vi "ZK HAL.vi"(11 "Interface":T1={"SYSTEM Interface"={"运行模式"=enum."维护模式", "站点类型"=enum."一体站", "CODMn类型"=enum."PLC版", "总磷总氮类型"=enum."单模块"}, "Pump Interface"={"Pump MB session in"=refnum}, "NH3N Interface"={"NH3N session in"=refnum, "氨氮自动测试量程配置"={"水样测试量程模式"=enum."AUTO", "空白核查量程模式"=enum."AUTO", "跨度核查量程模式"=enum."AUTO", "加标回收量程模式"=enum."AUTO"}}, "TP Interface"={"TP MB session in"=refnum, "总磷自动测试量程配置"={"水样测试量程模式"=enum."AUTO", "空白核查量程模式"=enum."AUTO", "跨度核查量程模式"=enum."AUTO", "加标回收量程模式"=enum."AUTO"}}, "TN Interface"={"TN MB session in"=refnum, "总氮自动测试量程配置"={"水样测试量程模式"=enum."AUTO", "空白核查量程模式"=enum."AUTO", "跨度核查量程模式"=enum."AUTO", "加标回收量程模式"=enum."AUTO"}}, "CODMn Interface"={"CODMn MB session in"=refnum, "CODMn自动测试量程配置"={"水样测试量程模式"=enum."AUTO", "空白核查量程模式"=enum."AUTO", "跨度核查量程模式"=enum."AUTO", "加标回收量程模式"=enum."AUTO"}}, "CODCr Interface"={"CODCr MB session in"=refnum, "CODCr自动测试量程配置"={"水样测试量程模式"=enum."AUTO", "空白核查量程模式"=enum."AUTO", "跨度核查量程模式"=enum."AUTO", "加标回收量程模式"=enum."AUTO"}}, "PLC_CODMn Interface"={"PLC版_CODMn状态"=0, "PLC版_CODMn测量数据区"={"因子编码"=0, "单位"=0, "标样参考值"=0.0, "水样数据时间"=timestamp(0 s since 1904-01-01), "水样实测值"=0.0, "水样数据标识"="", "标样数据时间"=timestamp(0 s since 1904-01-01), "标样实测值"=0.0, "标样数据标识"="", "空白数据时间"=timestamp(0 s since 1904-01-01), "空白实测值"=0.0, "空白数据标识"="", "零点核查数据时间"=timestamp(0 s since 1904-01-01), "零点核查实测值"=0.0, "零点核查数据标识"="", "跨度核查数据时间"=timestamp(0 s since 1904-01-01), "跨度核查实测值"=0.0, "跨度核查数据标识"="", "加标回收数据时间"=timestamp(0 s since 1904-01-01), "加标回收实测值"=0.0, "加标回收数据标识"="", "平行样数据时间"=timestamp(0 s since 1904-01-01), "平行样实测值"=0.0, "平行样数据标识"=""}}} {"PLC_CODMn Interface"."PLC版_CODMn状态" items=["待机", "润洗", "进样", "加草酸钠", "反滴定", "排液"]; "PLC_CODMn Interface"."PLC版_CODMn测量数据区"."单位" items=["ug/L", "mg/L", "ppm", "mg/m3", "cm", "ppb", "ug/m3", "%", "nmol/mol", "umol/mol", "MPN/L", "MPN/100ml", "ng/m3", "NTU", "无量纲", "ms/cm", "us/cm", "℃", "mV", "万个/L"]}) -> ()   [LabVIEW 2016]
uses:
  <vilib>/Plasmionique/MB Master/MB_Master/MB_Master.lvclass
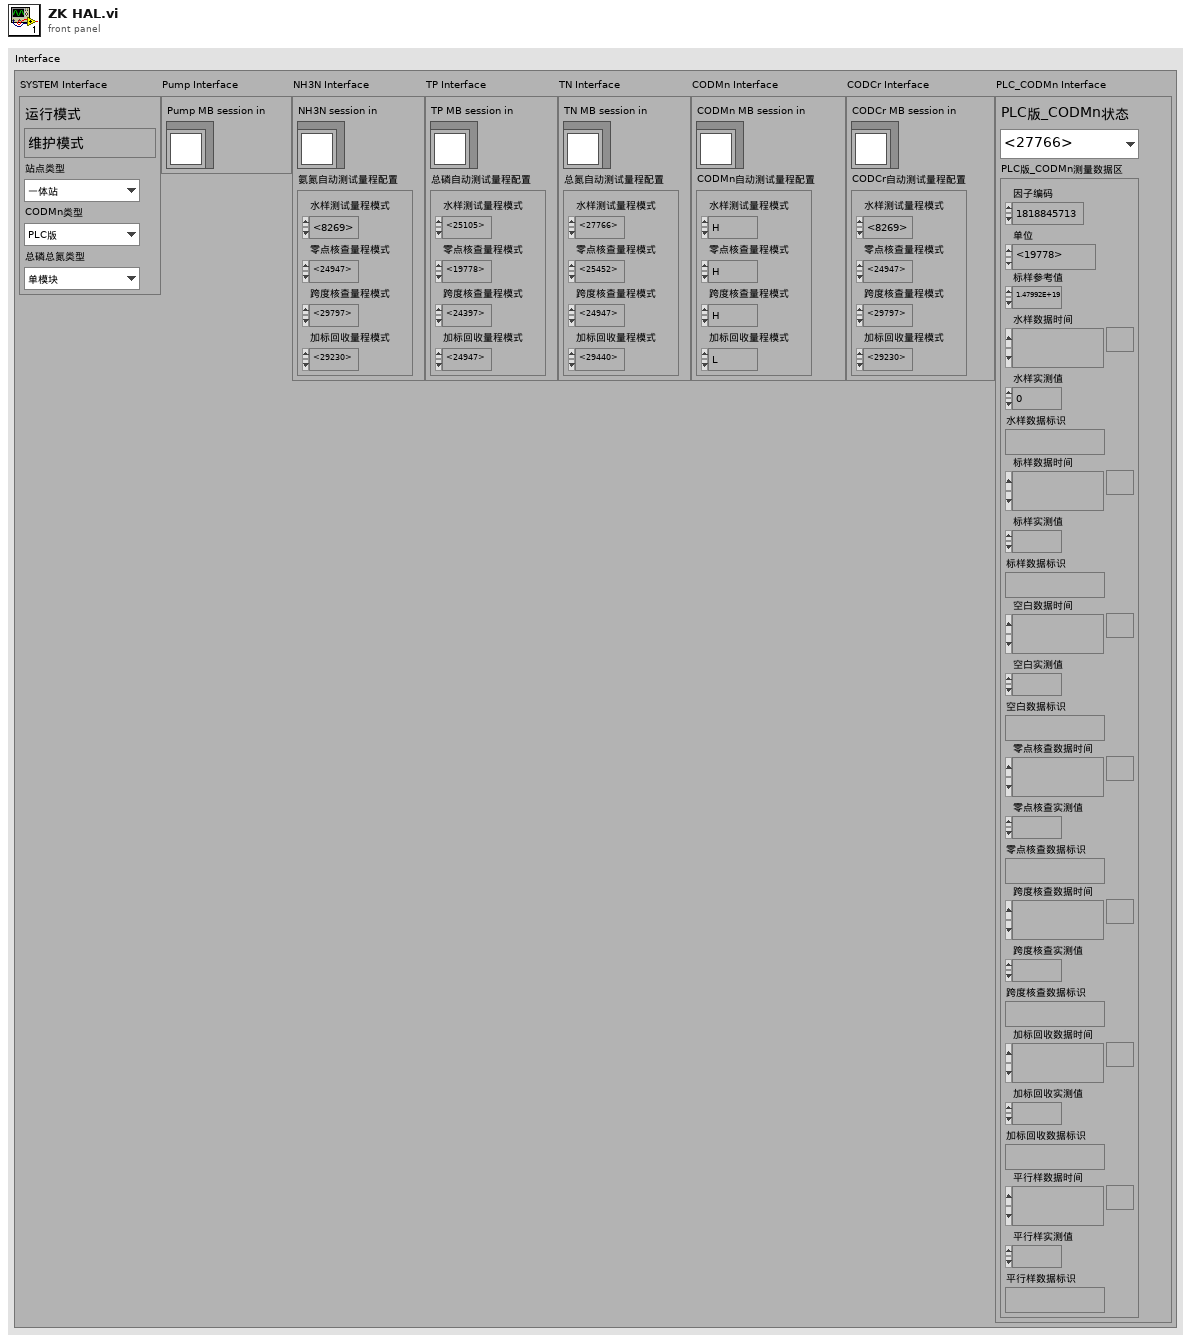
[diagram p1: front panel]
types:
  T1 = cluster{"SYSTEM Interface":cluster{"运行模式":enum16{"维护模式", "常规模式", "应急模式", "质控模式"}, "站点类型":enum16{"一体站", "固定站", "浮船"}, "CODMn类型":enum16{"PLC版", "单片机版"}, "总磷总氮类型":enum16{"单模块", "二合一模块"}}, "Pump Interface":cluster{"Pump MB session in":refnum<class "MB_Master.lvclass">}, "NH3N Interface":cluster{"NH3N session in":refnum<class "MB_Master.lvclass">, "氨氮自动测试量程配置":cluster{"水样测试量程模式":enum16{"H", "L", "AUTO"}, "空白核查量程模式":enum16{"H", "L", "AUTO"}, "跨度核查量程模式":enum16{"H", "L", "AUTO"}, "加标回收量程模式":enum16{"H", "L", "AUTO"}}}, "TP Interface":cluster{"TP MB session in":refnum<class "MB_Master.lvclass">, "总磷自动测试量程配置":cluster{"水样测试量程模式":enum16{"H", "L", "AUTO"}, "空白核查量程模式":enum16{"H", "L", "AUTO"}, "跨度核查量程模式":enum16{"H", "L", "AUTO"}, "加标回收量程模式":enum16{"H", "L", "AUTO"}}}, "TN Interface":cluster{"TN MB session in":refnum<class "MB_Master.lvclass">, "总氮自动测试量程配置":cluster{"水样测试量程模式":enum16{"H", "L", "AUTO"}, "空白核查量程模式":enum16{"H", "L", "AUTO"}, "跨度核查量程模式":enum16{"H", "L", "AUTO"}, "加标回收量程模式":enum16{"H", "L", "AUTO"}}}, "CODMn Interface":cluster{"CODMn MB session in":refnum<class "MB_Master.lvclass">, "CODMn自动测试量程配置":cluster{"水样测试量程模式":enum16{"H", "L", "AUTO"}, "空白核查量程模式":enum16{"H", "L", "AUTO"}, "跨度核查量程模式":enum16{"H", "L", "AUTO"}, "加标回收量程模式":enum16{"H", "L", "AUTO"}}}, "CODCr Interface":cluster{"CODCr MB session in":refnum<class "MB_Master.lvclass">, "CODCr自动测试量程配置":cluster{"水样测试量程模式":enum16{"H", "L", "AUTO"}, "空白核查量程模式":enum16{"H", "L", "AUTO"}, "跨度核查量程模式":enum16{"H", "L", "AUTO"}, "加标回收量程模式":enum16{"H", "L", "AUTO"}}}, "PLC_CODMn Interface":cluster{"PLC版_CODMn状态":u16, "PLC版_CODMn测量数据区":cluster{"因子编码":u32, "单位":u16, "标样参考值":sgl, "水样数据时间":timestamp, "水样实测值":sgl, "水样数据标识":string, "标样数据时间":timestamp, "标样实测值":sgl, "标样数据标识":string, "空白数据时间":timestamp, "空白实测值":sgl, "空白数据标识":string, "零点核查数据时间":timestamp, "零点核查实测值":sgl, "零点核查数据标识":string, "跨度核查数据时间":timestamp, "跨度核查实测值":sgl, "跨度核查数据标识":string, "加标回收数据时间":timestamp, "加标回收实测值":sgl, "加标回收数据标识":string, "平行样数据时间":timestamp, "平行样实测值":sgl, "平行样数据标识":string}}}
  T2 = cluster{"运行模式":enum16{"维护模式", "常规模式", "应急模式", "质控模式"}, "站点类型":enum16{"一体站", "固定站", "浮船"}, "CODMn类型":enum16{"PLC版", "单片机版"}, "总磷总氮类型":enum16{"单模块", "二合一模块"}}
  T3 = cluster{"Pump MB session in":refnum<class "MB_Master.lvclass">}
  T4 = cluster{"NH3N session in":refnum<class "MB_Master.lvclass">, "氨氮自动测试量程配置":cluster{"水样测试量程模式":enum16{"H", "L", "AUTO"}, "空白核查量程模式":enum16{"H", "L", "AUTO"}, "跨度核查量程模式":enum16{"H", "L", "AUTO"}, "加标回收量程模式":enum16{"H", "L", "AUTO"}}}
  T5 = cluster{"TP MB session in":refnum<class "MB_Master.lvclass">, "总磷自动测试量程配置":cluster{"水样测试量程模式":enum16{"H", "L", "AUTO"}, "空白核查量程模式":enum16{"H", "L", "AUTO"}, "跨度核查量程模式":enum16{"H", "L", "AUTO"}, "加标回收量程模式":enum16{"H", "L", "AUTO"}}}
  T6 = cluster{"TN MB session in":refnum<class "MB_Master.lvclass">, "总氮自动测试量程配置":cluster{"水样测试量程模式":enum16{"H", "L", "AUTO"}, "空白核查量程模式":enum16{"H", "L", "AUTO"}, "跨度核查量程模式":enum16{"H", "L", "AUTO"}, "加标回收量程模式":enum16{"H", "L", "AUTO"}}}
  T7 = cluster{"CODMn MB session in":refnum<class "MB_Master.lvclass">, "CODMn自动测试量程配置":cluster{"水样测试量程模式":enum16{"H", "L", "AUTO"}, "空白核查量程模式":enum16{"H", "L", "AUTO"}, "跨度核查量程模式":enum16{"H", "L", "AUTO"}, "加标回收量程模式":enum16{"H", "L", "AUTO"}}}
  T8 = cluster{"CODCr MB session in":refnum<class "MB_Master.lvclass">, "CODCr自动测试量程配置":cluster{"水样测试量程模式":enum16{"H", "L", "AUTO"}, "空白核查量程模式":enum16{"H", "L", "AUTO"}, "跨度核查量程模式":enum16{"H", "L", "AUTO"}, "加标回收量程模式":enum16{"H", "L", "AUTO"}}}
  T9 = cluster{"PLC版_CODMn状态":u16, "PLC版_CODMn测量数据区":cluster{"因子编码":u32, "单位":u16, "标样参考值":sgl, "水样数据时间":timestamp, "水样实测值":sgl, "水样数据标识":string, "标样数据时间":timestamp, "标样实测值":sgl, "标样数据标识":string, "空白数据时间":timestamp, "空白实测值":sgl, "空白数据标识":string, "零点核查数据时间":timestamp, "零点核查实测值":sgl, "零点核查数据标识":string, "跨度核查数据时间":timestamp, "跨度核查实测值":sgl, "跨度核查数据标识":string, "加标回收数据时间":timestamp, "加标回收实测值":sgl, "加标回收数据标识":string, "平行样数据时间":timestamp, "平行样实测值":sgl, "平行样数据标识":string}}
  T10 = cluster{"水样测试量程模式":enum16{"H", "L", "AUTO"}, "空白核查量程模式":enum16{"H", "L", "AUTO"}, "跨度核查量程模式":enum16{"H", "L", "AUTO"}, "加标回收量程模式":enum16{"H", "L", "AUTO"}}
  T11 = cluster{"因子编码":u32, "单位":u16, "标样参考值":sgl, "水样数据时间":timestamp, "水样实测值":sgl, "水样数据标识":string, "标样数据时间":timestamp, "标样实测值":sgl, "标样数据标识":string, "空白数据时间":timestamp, "空白实测值":sgl, "空白数据标识":string, "零点核查数据时间":timestamp, "零点核查实测值":sgl, "零点核查数据标识":string, "跨度核查数据时间":timestamp, "跨度核查实测值":sgl, "跨度核查数据标识":string, "加标回收数据时间":timestamp, "加标回收实测值":sgl, "加标回收数据标识":string, "平行样数据时间":timestamp, "平行样实测值":sgl, "平行样数据标识":string}
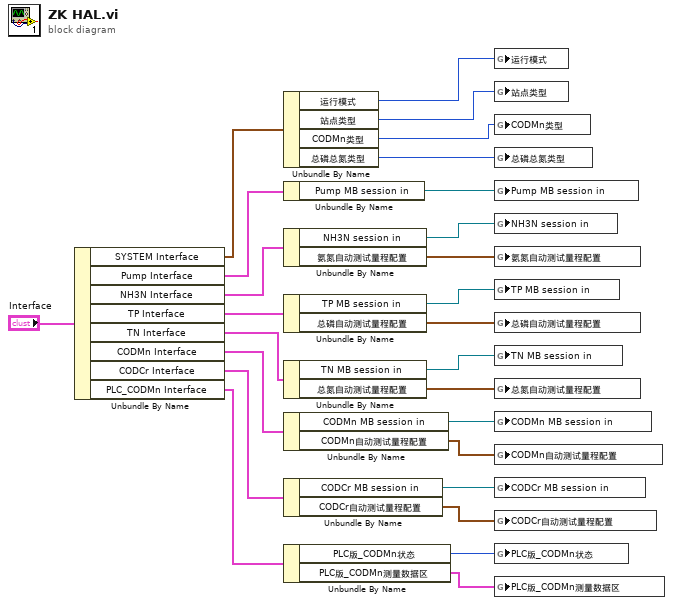
[diagram p0: block diagram]
diagram:
  n1 = Unbundle By Name("Interface") -> ("SYSTEM Interface"=w25:T2, "Pump Interface"=w23:T3, "NH3N Interface"=w21:T4, "TP Interface"=w18:T5, "TN Interface"=w15:T6, "CODMn Interface"=w12:T7, "CODCr Interface"=w9:T8, "PLC_CODMn Interface"=w6:T9)
  n2 = Unbundle By Name(w25) -> ("运行模式"=w24:enum16{"维护模式", "常规模式", "应急模式", "质控模式"}, "站点类型"=w2:enum16{"一体站", "固定站", "浮船"}, "CODMn类型"=w3:enum16{"PLC版", "单片机版"}, "总磷总氮类型"=w1:enum16{"单模块", "二合一模块"})
  n3 = Unbundle By Name(w23) -> ("Pump MB session in"=w22:refnum<class "MB_Master.lvclass">)
  n4 = Unbundle By Name(w21) -> ("NH3N session in"=w19:refnum<class "MB_Master.lvclass">, "氨氮自动测试量程配置"=w20:T10)
  n5 = Unbundle By Name(w18) -> ("TP MB session in"=w17:refnum<class "MB_Master.lvclass">, "总磷自动测试量程配置"=w16:T10)
  n6 = Unbundle By Name(w15) -> ("TN MB session in"=w14:refnum<class "MB_Master.lvclass">, "总氮自动测试量程配置"=w13:T10)
  n7 = Unbundle By Name(w12) -> ("CODMn MB session in"=w11:refnum<class "MB_Master.lvclass">, "CODMn自动测试量程配置"=w10:T10)
  n8 = Unbundle By Name(w9) -> ("CODCr MB session in"=w8:refnum<class "MB_Master.lvclass">, "CODCr自动测试量程配置"=w7:T10)
  n9 = Unbundle By Name(w6) -> ("PLC版_CODMn状态"=w5:u16, "PLC版_CODMn测量数据区"=w4:T11)
  n10 = global write "系统交互.vi" "运行模式"(w24) -> ()
  n11 = global write "系统交互.vi" "站点类型"(w2) -> ()
  n12 = global write "系统交互.vi" "CODMn类型"(w3) -> ()
  n13 = global write "系统交互.vi" "总磷总氮类型"(w1) -> ()
  n14 = global write "系统交互.vi" "Pump MB session in"(w22) -> ()
  n15 = global write "系统交互.vi" "NH3N session in"(w19) -> ()
  n16 = global write "系统交互.vi" "氨氮自动测试量程配置"(w20) -> ()
  n17 = global write "系统交互.vi" "TP MB session in"(w17) -> ()
  n18 = global write "系统交互.vi" "总磷自动测试量程配置"(w16) -> ()
  n19 = global write "系统交互.vi" "TN MB session in"(w14) -> ()
  n20 = global write "系统交互.vi" "总氮自动测试量程配置"(w13) -> ()
  n21 = global write "系统交互.vi" "CODMn MB session in"(w11) -> ()
  n22 = global write "系统交互.vi" "CODMn自动测试量程配置"(w10) -> ()
  n23 = global write "系统交互.vi" "CODCr MB session in"(w8) -> ()
  n24 = global write "系统交互.vi" "CODCr自动测试量程配置"(w7) -> ()
  n25 = global write "系统交互.vi" "PLC版_CODMn状态"(w5) -> ()
  n26 = global write "系统交互.vi" "PLC版_CODMn测量数据区"(w4) -> ()
